vi "Math.Convert Ratio to other Units.vi"(8 "error in (no error)":errorcluster, 10 "ratio units":enum16{"dB", "linear ratio", "%"}(ring), 11 "linear ratio":dbl format="%.3e") -> (0 "error out":errorcluster, 2 "unit label":string, 3 "converted ratio":dbl format="%.3e")   [LabVIEW 2018]
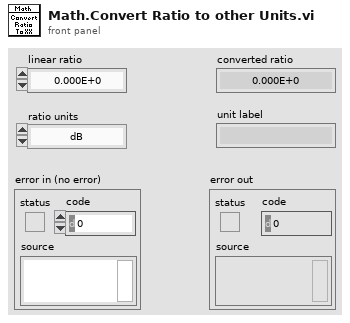
[diagram p1: front panel]
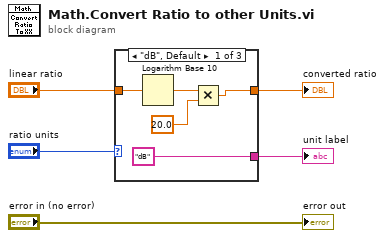
[diagram p0: block diagram]
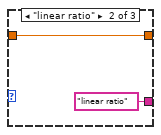
[diagram p2: hidden frame]
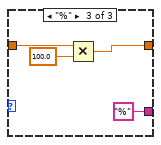
[diagram p3: hidden frame]
diagram:
  n1 = case shown="\"dB\", Default" "ratio units" {
    tunnel: [w7 w12 w14] -> w3
    tunnel: "linear ratio" -> [w10 w12 w16]
    tunnel: ["dB" "linear ratio" "%"] -> w2
    frame "dB", Default {
      n2 = Logarithm Base 10(1:w10) -> (0:w9:dbl)
      n3 = Multiply(x=w9, y=20.0) -> (x*y=w7:dbl)
    }
    frame "linear ratio" {
    }
    frame "%" {
      n4 = Multiply(x=w16, y=100.0) -> (x*y=w14:dbl)
    }
  }
  "converted ratio" <- w3
  "unit label" <- w2
  "error out" <- "error in (no error)"
